vi "Serial_Read.vi"(8 "error in (no error)":errorcluster, 9 "Bytes":i32, 11 "Python in":cluster{"Python":refnum<k35>, "py file":path}) -> (0 "error out":errorcluster, 1 "text read":string, 3 "Python out":cluster{"Python":refnum<k35>, "py file":path})   [LabVIEW 2020]
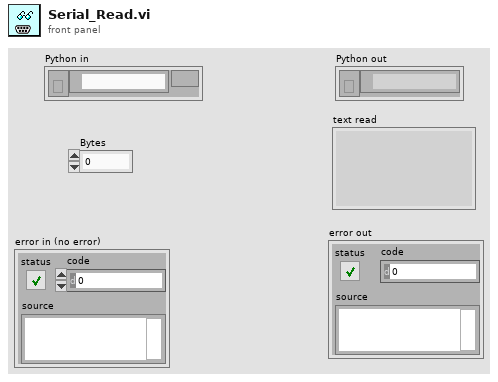
[diagram p1: front panel]
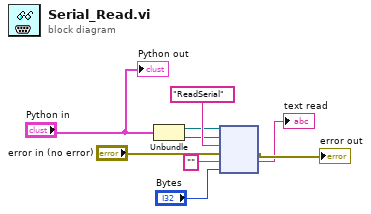
[diagram p0: block diagram]
diagram:
  n1 = Unbundle("Python in") -> ("Python"=w5:refnum<k35>, "py file"=w4:path)
  n2 = node(w5, w4, "ReadSerial" ("function name"), "error in (no error)", "" ("function name"), "Bytes") -> (→"error out":errorcluster, →"text read":string)  [unwired: 1 in, 3 out]
  "Python out" <- "Python in"
